vi "Connector 2 DO Engine Sim 2.vi"(11 "Packet":u64) -> ()   [LabVIEW 2014]
uses:
  <vilib>/rvi/eio/common/nirviEmuTemplateMethod_errors.vi
  <vilib>/eio/EIONode/EIONode.xnode
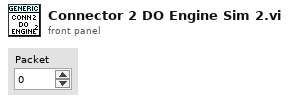
[diagram p1: front panel]
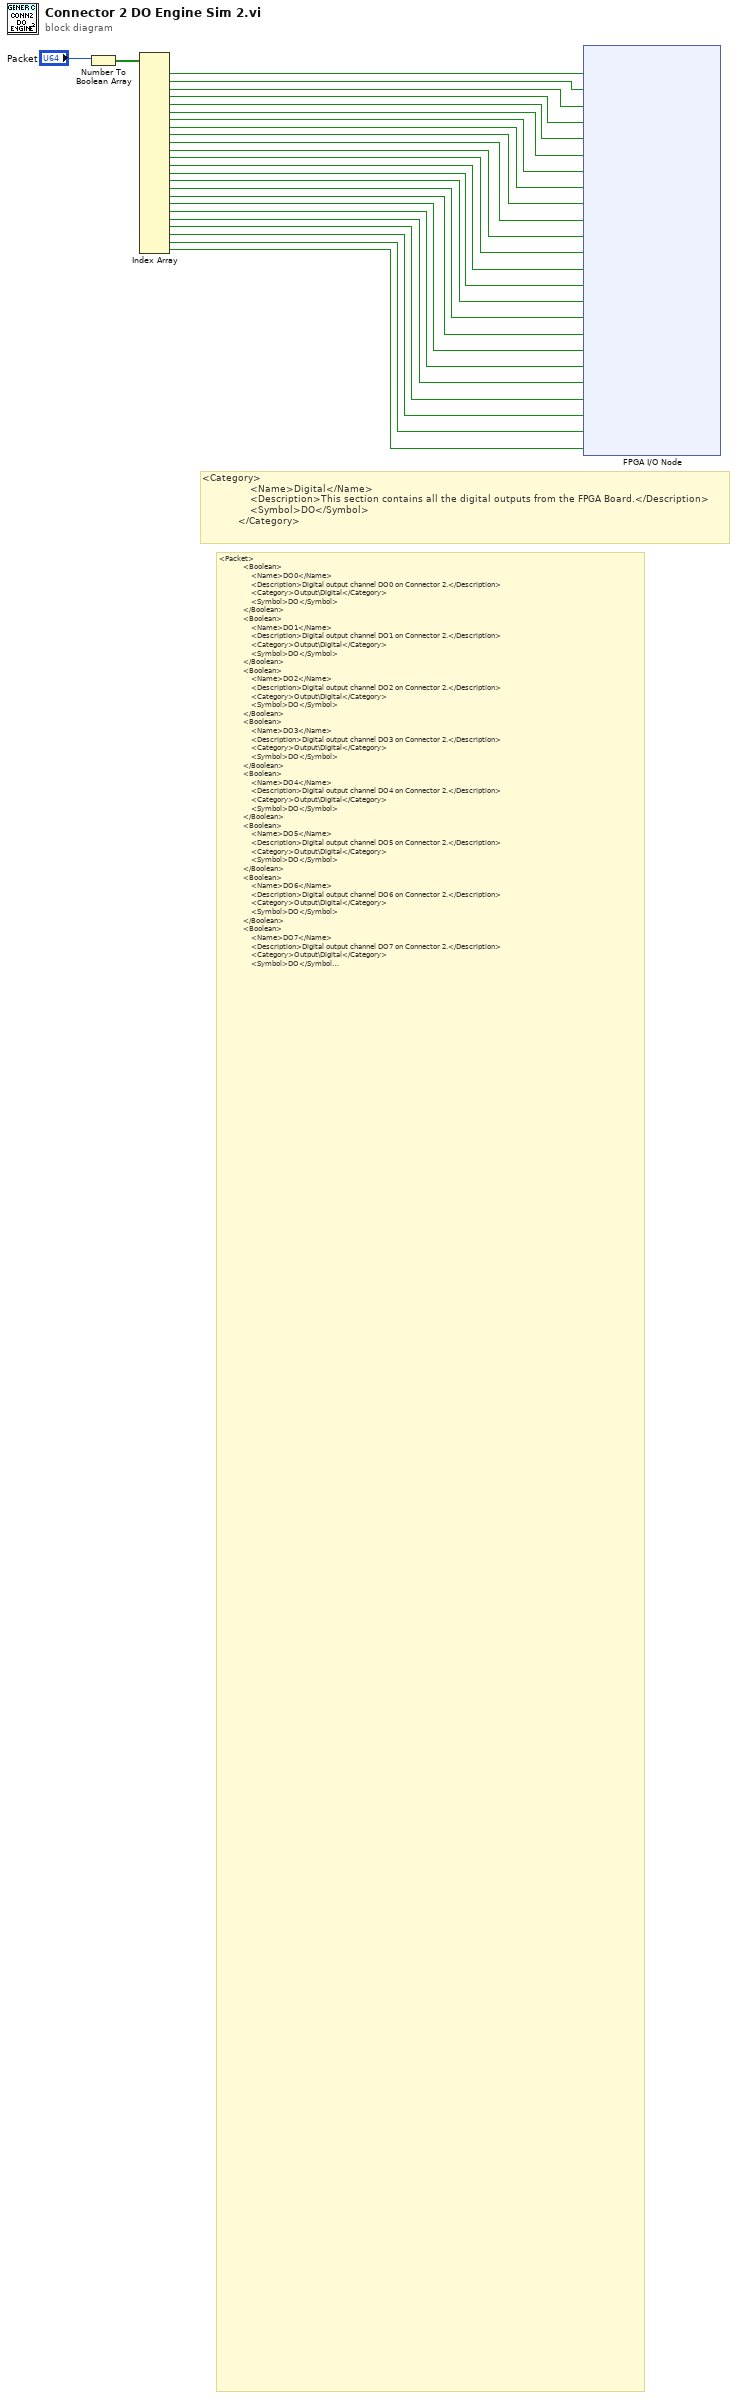
[diagram p0: block diagram]
diagram:
  # "<Packet>\n            <Boolean>\n                <Name>DO0</Name>\n                <Description>Digital output channel DO0 on Connector 2.</Description>\n                <Category>Output\\Digital</Category>\n                <Symbol>DO</Symbol>\n            </Boolean>\n            <Boolean>\n                <Name>DO1</Name>\n                <Description>Digital output channel DO1 on Connector 2.</Description>\n                <Category>Output\\Digital</Category>\n                <Symbol>DO</Symbol>\n            </Boolean>\n            <Boolean>\n                <Name>DO2</Name>\n                <Description>Digital output channel DO2 on Connector 2.</Description>\n                <Category>Output\\Digital</Category>\n                <Symbol>DO</Symbol>\n            </Boolean>\n            <Boolean>\n                <Name>DO3</Name>\n                <Description>Digital output channel DO3 on Connector 2.</Description>\n                <Category>Output\\Digital</Category>\n                <Symbol>DO</Symbol>\n            </Boolean>\n            <Boolean>\n                <Name>DO4</Name>\n                <Description>Digital output channel DO4 on Connector 2.</Description>\n                <Category>Output\\Digital</Category>\n                <Symbol>DO</Symbol>\n            </Boolean>\n            <Boolean>\n                <Name>DO5</Name>\n                <Description>Digital output channel DO5 on Connector 2.</Description>\n                <Category>Output\\Digital</Category>\n                <Symbol>DO</Symbol>\n            </Boolean>\n            <Boolean>\n                <Name>DO6</Name>\n                <Description>Digital output channel DO6 on Connector 2.</Description>\n                <Category>Output\\Digital</Category>\n                <Symbol>DO</Symbol>\n            </Boolean>\n            <Boolean>\n                <Name>DO7</Name>\n                <Description>Digital output channel DO7 on Connector 2.</Description>\n                <Category>Output\\Digital</Category>\n                <Symbol>DO</Symbol>\n            </Boolean>\n             <Boolean>\n                <Name>DO8</Name>\n                <Description>Digital output channel DO8 on Connector 2.</Description>\n                <Category>Output\\Digital</Category>\n                <Symbol>DO</Symbol>\n            </Boolean>\n            <Boolean>\n                <Name>DO9</Name>\n                <Description>Digital output channel DO9 on Connector 2.</Description>\n                <Category>Output\\Digital</Category>\n                <Symbol>DO</Symbol>\n            </Boolean>\n            <Boolean>\n                <Name>DO10</Name>\n                <Description>Digital output channel DO10 on Connector 2.</Description>\n                <Category>Output\\Digital</Category>\n                <Symbol>DO</Symbol>\n            </Boolean>\n            <Boolean>\n                <Name>DO11</Name>\n                <Description>Digital output channel DO11 on Connector 2.</Description>\n                <Category>Output\\Digital</Category>\n                <Symbol>DO</Symbol>\n            </Boolean>\n            <Boolean>\n                <Name>DO12</Name>\n                <Description>Digital output channel DO12 on Connector 2.</Description>\n                <Category>Output\\Digital</Category>\n                <Symbol>DO</Symbol>\n            </Boolean>\n            <Boolean>\n                <Name>DO13</Name>\n                <Description>Digital output channel DO13 on Connector 2.</Description>\n                <Category>Output\\Digital</Category>\n                <Symbol>DO</Symbol>\n            </Boolean>\n            <Boolean>\n                <Name>DO14</Name>\n                <Description>Digital output channel DO14 on Connector 2.</Description>\n                <Category>Output\\Digital</Category>\n                <Symbol>DO</Symbol>\n            </Boolean>\n            <Boolean>\n                <Name>DO15</Name>\n                <Description>Digital output channel DO15 on Connector 2.</Description>\n                <Category>Output\\Digital</Category>\n                <Symbol>DO</Symbol>\n            </Boolean>\n            <Boolean>\n                <Name>Key Switch</Name>\n                <Description>Digital output channel DO16 on Connector 2.</Description>\n                <Category>Output\\Digital</Category>\n                <Symbol>DO</Symbol>\n            </Boolean>\n            <Boolean>\n                <Name>DO34</Name>\n                <Description>Digital output channel DO34 on Connector 2.</Description>\n                <Category>Output\\Digital</Category>\n                <Symbol>DO</Symbol>\n            </Boolean>\n            <Boolean>\n                <Name>DO36</Name>\n                <Description>Digital output channel DO36 on Connector 2.</Description>\n                <Category>Output\\Digital</Category>\n                <Symbol>DO</Symbol>\n            </Boolean>\n            <Boolean>\n                <Name>DO38</Name>\n                <Description>Digital output channel DO38 on Connector 2.</Description>\n                <Category>Output\\Digital</Category>\n                <Symbol>DO</Symbol>\n            </Boolean>\n            <Boolean>\n                <Name>DO39</Name>\n                <Description>Digital output channel DO39 on Connector 2.</Description>\n                <Category>Output\\Digital</Category>\n                <Symbol>DO</Symbol>\n            </Boolean>\n        </Packet>"
  # "<Category>\n                <Name>Digital</Name>\n                <Description>This section contains all the digital outputs from the FPGA Board.</Description>\n                <Symbol>DO</Symbol>\n            </Category>"
  n1 = Number To Boolean Array(number="Packet") -> (Boolean array=w25:bool[])
  n2 = Index Array(array=w25) -> (element #1=w24:bool, element #2=w23:bool, element #3=w22:bool, element #4=w21:bool, element #5=w20:bool, element #6=w19:bool, element #7=w18:bool, element #8=w17:bool, element #9=w16:bool, element #10=w15:bool, element #11=w14:bool, element #12=w13:bool, element #13=w12:bool, element #14=w11:bool, element #15=w10:bool, element #16=w9:bool, element #17=w8:bool, element #18=w7:bool, element #19=w6:bool, element #20=w5:bool, element #21=w4:bool, element #22=w3:bool, element #23=w2:bool, element #24=w1:bool)  [unwired: 24 in]
  n3 = xnode "FPGA I/O Node"("Connector2/DIO0"=w24, "Connector2/DIO1"=w23, "Connector2/DIO2"=w22, "Connector2/DIO3"=w21, "Connector2/DIO4"=w20, "Connector2/DIO5"=w19, "Connector2/DIO6"=w18, "Connector2/DIO7"=w17, "Connector2/DIO8"=w16, "Connector2/DIO9"=w15, "Connector2/DIO10"=w14, "Connector2/DIO11"=w13, "Connector2/DIO12"=w12, "Connector2/DIO13"=w11, "Connector2/DIO14"=w10, "Connector2/DIO15"=w9, "Key Switch"=w8, "Connector2/DIO30"=w7, "Connector2/DIO32"=w6, "Connector2/DIO34"=w5, "Connector2/DIO36"=w4, "Connector2/DIO37"=w3, "Connector2/DIO38"=w2, "Connector2/DIO39"=w1) -> ()  [unwired: 24 in, 24 out]
